vi "ReadCalibrationFilesSingle.vi"(8 "error in (no error)":errorcluster, 11 "MagSpecCamera in":refnum<class "MagSpecCamera.lvclass">) -> (0 "error out":errorcluster, 3 "MagSpecCamera in":refnum<class "MagSpecCamera.lvclass">)   [LabVIEW 2020, in "MagSpecCamera.lvclass"]
uses:
  MagSpecCamera.lvclass
  MagSpecCamera.lvclass/MagSpecCamera.ctl
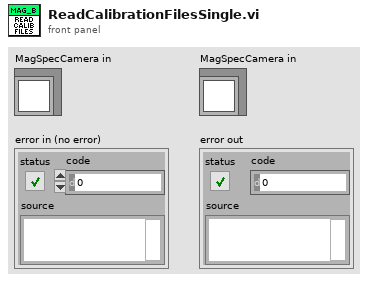
[diagram p1: front panel]
types:
  T1 = typedef "OnOffTypeDef.ctl" = enum16{"off", "on"}
  T2 = typedef "CalibrationCluster.ctl" = cluster{"bending angle Front":dbl[], "bending angle Side":dbl[], "screen [m] Front":dbl[], "screen [m] Side":dbl[], "momentum [MeV/c]":dbl[], "total path [m]":dbl[], "x[mm](rms)":dbl[], "x[mm](rms,b)":dbl[], "y[mm](rms)":dbl[], "y[mm](rms,b)":dbl[]}
  T3 = typedef "CameraSettings_File.ctl" = cluster{"FOV [mm]":dbl, "Left edge [mm]":dbl, "ROI Y offset":dbl, "ROI height":dbl, "ROI X offset":dbl, "ROI width":dbl, "Y center pixel":dbl, "Y Start":dbl, "Y End":dbl, "X Start":dbl, "X End":dbl, "rot [deg]":dbl}
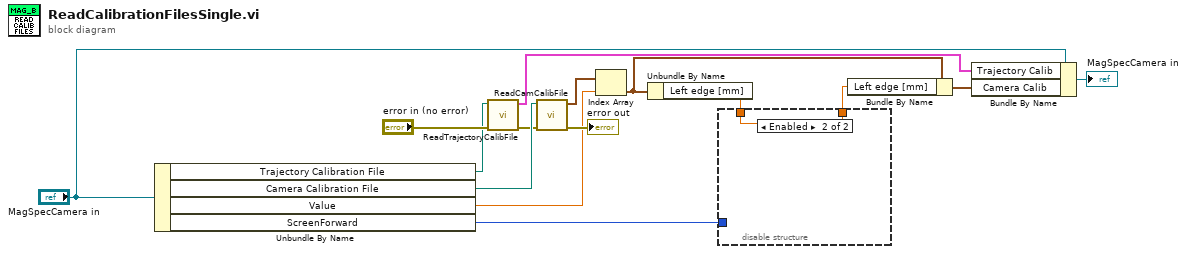
[diagram p0: block diagram]
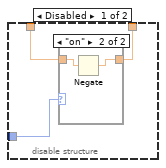
[diagram p2: hidden frame]
diagram:
  n1 = Unbundle By Name("MagSpecCamera in") -> ("Trajectory Calibration File"=w8:path, "Camera Calibration File"=w11:path, "Value"=w6:dbl, "ScreenForward"=w5:T1)
  n2 = call "ReadTrajectoryCalibFile.vi"("error in (no error)"="error in (no error)", "Spec_Calib_file in"=w8) -> ("error out"=w10:errorcluster, "Cluster"=w13:T2)  [unwired: 8 in]
  n3 = call "ReadCamCalibFile.vi"("error in (no error)"=w10, "Spec_Calib_file in"=w11) -> ("error out"=→"error out":errorcluster, "Cam Calib Array"=w7:T3[])  [unwired: 8 in]
  n4 = Index Array(array=w7, index=w6) -> (element=w3:T3)
  n5 = Unbundle By Name(w3) -> ("Left edge [mm]"=w4:dbl)
  n6 = disable-structure shown="Enabled" {
    disable-tunnel: w5 -> [w18 _]
    disable-tunnel: w4 -> [w17 w22]
    disable-tunnel: [w16 w22] -> w1
    frame Disabled {
      n7 = case shown="\"on\"" w18 {
        tunnel: w17 -> [w19 w21]
        tunnel: [w19 w20] -> w16
        frame "off", Default {
        }
        frame "on" {
          n8 = Negate(x=w21) -> (-x=w20:dbl)
        }
      }
    }
    frame Enabled {
    }
  }
  n9 = Bundle By Name(cluster=w3, "Left edge [mm]"=w1) -> (w2:T3)
  n10 = Bundle By Name(cluster="MagSpecCamera in", "Trajectory Calib"=w13, "Camera Calib"=w2) -> (→"MagSpecCamera in":refnum<class "MagSpecCamera.lvclass">)
